vi "setDevicePara.vi"(8 "error in (no error)":errorcluster, 11 "Acquisition Parameters 2":T1={"Camera "=FALSE, "Voltage stimulus"=FALSE, "Period [ms]"=200.0, "Duration [ms]"=0.2, "Delay [ms]"=0.0, "Pulses [#]"=10, "Vhold [mV]"=50.0, "Vpulse [mV]"=0.0, "Vstep [mV]"=10.0, "N"=10, "Thold [ms]"=0.0, "Tpulse [ms]"=200.0, "sampling rate [kHz]"="1,25", "current range [nA]"="20", "time [s]"=2.0} {"Tpulse [ms]" format="%_5f"; "Thold [ms]" format="%_5f"; "Vstep [mV]" format="%_5f"; "Vpulse [mV]" format="%_5f"; "Vhold [mV]" format="%_5f"; "Delay [ms]" format="%_5f"; "Duration [ms]" format="%_5f"; "Period [ms]" format="%_5f"}) -> (0 "error out":errorcluster, 3 "function return":u32(ring))   [LabVIEW 2021]
uses:
  <userlib>/er4commlib_labview/er4commlib_labview.lvlib
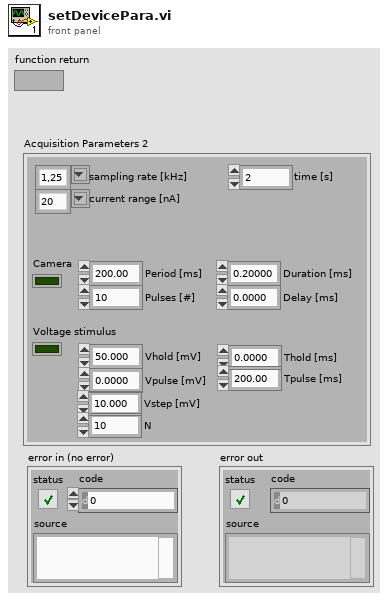
[diagram p1: front panel]
types:
  T1 = cluster{"Camera ":bool, "Voltage stimulus":bool, "Period [ms]":dbl, "Duration [ms]":dbl, "Delay [ms]":dbl, "Pulses [#]":u32, "Vhold [mV]":dbl, "Vpulse [mV]":dbl, "Vstep [mV]":dbl, "N":u32, "Thold [ms]":dbl, "Tpulse [ms]":dbl, "sampling rate [kHz]":string, "current range [nA]":string, "time [s]":dbl}
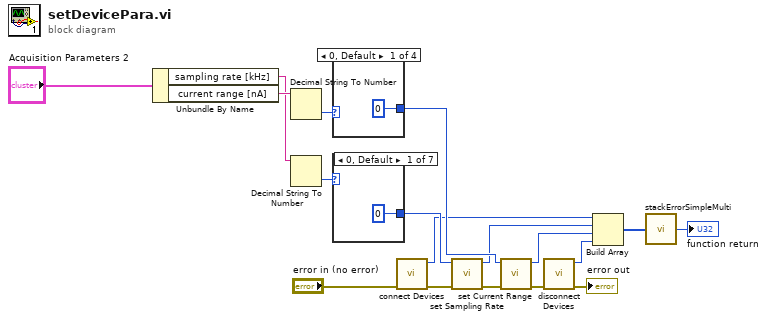
[diagram p0: block diagram]
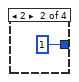
[diagram p2: hidden frame]
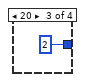
[diagram p3: hidden frame]
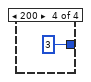
[diagram p4: hidden frame]
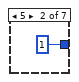
[diagram p5: hidden frame]
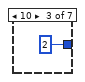
[diagram p6: hidden frame]
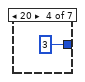
[diagram p7: hidden frame]
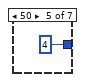
[diagram p8: hidden frame]
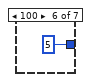
[diagram p9: hidden frame]
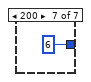
[diagram p10: hidden frame]
diagram:
  n1 = Unbundle By Name("Acquisition Parameters 2") -> ("sampling rate [kHz]"=w12:string, "current range [nA]"=w15:string)
  n2 = Decimal String To Number(string=w15) -> (number=w16:i32)  [unwired: 2 in, 1 out]
  n3 = Decimal String To Number(string=w12) -> (number=w13:i32)  [unwired: 2 in, 1 out]
  n4 = case shown="0, Default" w16 {
    tunnel: [0 1 2 3] -> w17
    frame 0, Default {
    }
    frame 2 {
    }
    frame 20 {
    }
    frame 200 {
    }
  }
  n5 = case shown="0, Default" w13 {
    tunnel: [0 1 2 3 4 5 6] -> w14
    frame 0, Default {
    }
    frame 5 {
    }
    frame 10 {
    }
    frame 20 {
    }
    frame 50 {
    }
    frame 100 {
    }
    frame 200 {
    }
  }
  n6 = call <userlib>:"connect Devices.vi"("error in (no error)"="error in (no error)") -> ("error out"=w5:errorcluster, "function return"=w1:u32)  [unwired: 9 in]
  n7 = call <userlib>:"set Sampling Rate.vi"("error in (no error)"=w5, "samplingRateIdx"=w14) -> ("error out"=w18:errorcluster, "function return"=w11:u32)  [unwired: 8 in]
  n8 = call <userlib>:"set Current Range.vi"("error in (no error)"=w18, "currentRangeIdx"=w17) -> ("error out"=w4:errorcluster, "function return"=w10:u32)  [unwired: 8 in]
  n9 = call <userlib>:"disconnect Devices.vi"("error in (no error)"=w4) -> ("error out"=→"error out":errorcluster, "function return"=w2:u32)  [unwired: 9 in]
  n10 = Build Array(w1, w11, w10, w2) -> (w9:u32[])
  n11 = call "stackErrorSimpleMulti.vi"("Error List"=w9) -> ("Error Out"=→"function return":u32)
